vi "macro_LTV_Unicycle_Ctrl_TrajSample_Execute.vi"() -> ()   [LabVIEW 2019, in "Trajectory_Library.lvlib"]
uses:
  Trajectory_Library.lvlib
  TypeDef/CHASSIS_SPEEDS.ctl
  TypeDef/POSE2D.ctl
  TypeDef/TRANSLATION2D.ctl
  TypeDef/ROTATION2D.ctl
  TypeDef/TRAJ_STATE.ctl
panel:
  in  "TRAJ_STATE":T1={"TimeSeconds"=0.0, "Velocity"=0.0, "Acceleration"=0.0, "POSE"={"TRANSLATION"={"X"=0.0, "Y"=0.0}, "ROTATION"={"VALUE"=0.0, "COS"=1.0, "SIN"=0.0}}, "Curvature"=0.0} {"POSE"."ROTATION"."SIN" format="%13.4f"; "POSE"."ROTATION"."COS" format="%13.4f"; "POSE"."ROTATION"."VALUE" format="%13.4f"; "POSE"."TRANSLATION"."Y" format="%14.3f"; "POSE"."TRANSLATION"."X" format="%14.3f"}
  in  "CurrentPose":T2={"TRANSLATION"={"X"=0.0, "Y"=0.0}, "ROTATION"={"VALUE"=0.0, "COS"=1.0, "SIN"=0.0}} {"ROTATION"."SIN" format="%13.4f"; "ROTATION"."COS" format="%13.4f"; "ROTATION"."VALUE" format="%13.4f"; "TRANSLATION"."Y" format="%14.3f"; "TRANSLATION"."X" format="%14.3f"}
  out "ChassisSpeeds":T5 {"vOmega" format="%10.3f"; "vY" format="%10.3f"; "vX" format="%10.3f"}
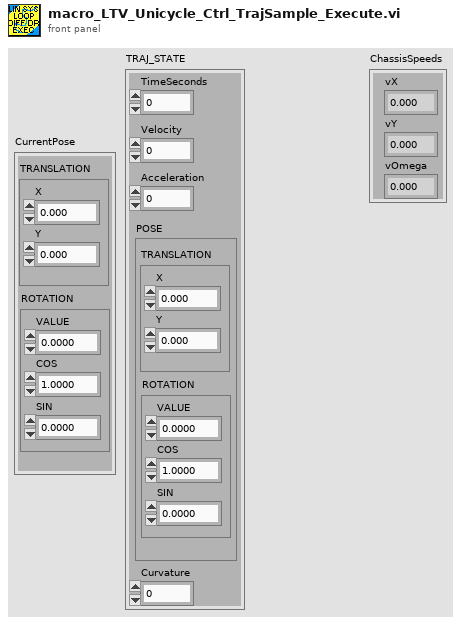
[diagram p1: front panel]
types:
  T1 = typedef "Trajectory_Library.lvlib/TRAJ_STATE.ctl" = cluster{"TimeSeconds":dbl, "Velocity":dbl, "Acceleration":dbl, "POSE":T2, "Curvature":dbl}
  T2 = typedef "Trajectory_Library.lvlib/POSE2D.ctl" = cluster{"TRANSLATION":T3, "ROTATION":T4}
  T3 = typedef "Trajectory_Library.lvlib/TRANSLATION2D.ctl" = cluster{"X":dbl, "Y":dbl}
  T4 = typedef "Trajectory_Library.lvlib/ROTATION2D.ctl" = cluster{"VALUE":dbl, "COS":dbl, "SIN":dbl}
  T5 = typedef "Trajectory_Library.lvlib/CHASSIS_SPEEDS.ctl" = cluster{"vX":dbl, "vY":dbl, "vOmega":dbl}
  T6 = typedef "LTV_UNICYCLE_CONTROLLER_MODEL_PARAMS.CTL" = cluster{"Max linear ctrl effort M/S":dbl, "Max angular ctrl effort Rad/S":dbl, "Max Heading Meas Tol Rad":dbl, "Max X Pos Meas Tol M":dbl, "Max Y Pos Meas Tol M":dbl, "Max Linear Vel M/S":dbl}
  T7 = typedef "LTV_UNICYCLE_CONTROLLER_TOLERANCE.CTL" = cluster{"Max Heading Tolerance Rad":dbl, "Max X Tolerance M":dbl, "Max Y Tolerance M":dbl}
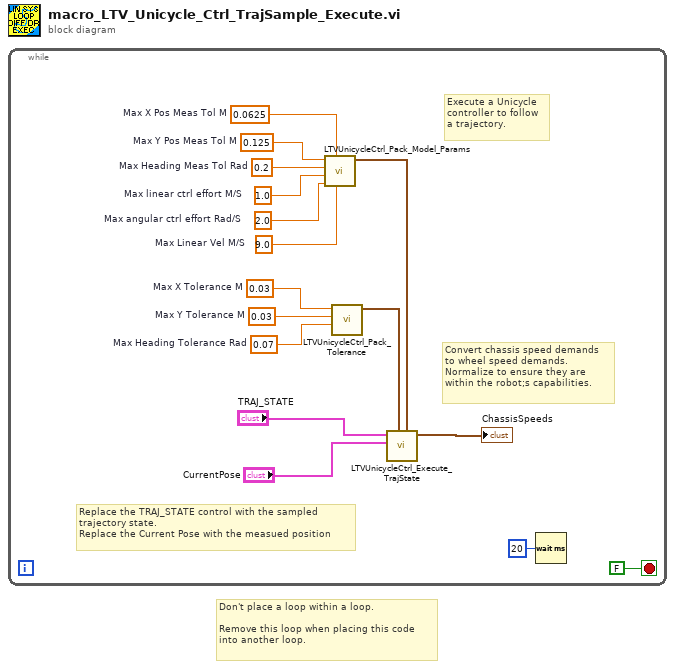
[diagram p0: block diagram]
diagram:
  # "Don't place a loop within a loop.\n \nRemove this loop when placing this code\ninto another loop."
  n1 = while {
    stop <- FALSE stop-if-true
    w4 = 0.03  # Max X Tolerance M
    w5 = 0.03  # Max Y Tolerance M
    w6 = 0.07  # Max Heading Tolerance Rad
    w7 = 0.125  # Max Y Pos Meas Tol M
    w8 = 0.2  # Max Heading Meas Tol Rad
    w9 = 1.0  # Max linear ctrl effort M/S
    w10 = 2.0  # Max angular ctrl effort Rad/S
    w11 = 0.0625  # Max X Pos Meas Tol M
    w12 = 9.0  # Max Linear Vel M/S
    # "Convert chassis speed demands\nto wheel speed demands.   \nNormalize to ensure they are \nwithin the robot;s capabilities."
    # "Replace the TRAJ_STATE control with the sampled \ntrajectory state.\nReplace the Current Pose with the measued position"
    # "Execute a Unicycle\ncontroller to follow\na trajectory."
    n2 = call "LTVUnicycleCtrl_Pack_Model_Params.vi"("Max Linear Vel M/S"=w12, "Max X Pos Meas Tol M"=w11, "Max angular ctrl effort Rad/S"=w10, "Max linear ctrl effort M/S"=w9, "Max Heading Meas Tol Rad"=w8, "Max Y Pos Meas Tol M"=w7) -> ("LTV_Unicycle_Ctrl_Model _Params"=w13:T6)  [unwired: 5 in]
    n3 = call "LTVUnicycleCtrl_Pack_Tolerance.vi"("Max Heading Tolerance Rad"=w6, "Max Y Tolerance M"=w5, "Max X Tolerance M"=w4) -> ("LTV_Unicycle_Ctrl_Tolerance"=w14:T7)  [unwired: 8 in]
    n4 = call "LTVUnicycleCtrl_Execute_TrajState.vi"("LTV_Unicycle_Ctrl_Model"=w13, "LTV_Unicycle_Ctrl_Tolerance"=w14, "CurrentPose"="CurrentPose", "TRAJ_STATE"="TRAJ_STATE") -> ("ChassisSpeeds"=→"ChassisSpeeds":T5)  [unwired: 4 in, 3 out]
    n5 = Wait (ms)(milliseconds to wait=u32 20) -> ()  [unwired: 1 out]
  }
